vi "setEndLabel.vi"(0 "reference":refnum<class "SegmentedLineEdge.lvclass">, 1 "endLabel":string, 5 "error in (no error)":errorcluster) -> (14 "reference out":refnum<class "SegmentedLineEdge.lvclass">, 19 "error out":errorcluster)   [LabVIEW 2016, in "SegmentedLineEdge.lvclass"]
doc: "public void setEndLabel(String newValue)"
uses:
  <resource>/Framework/Providers/Open_GDS/UML/SegmentedLineEdge_class/SegmentedLineEdge.lvclass
panel:
  # "Always set\nVI Server class\nto current VI. Do not\nconnect this control\nto the connector pane.\n(Tip!: Just drag\nand drop the icon\ninto the refnum)"
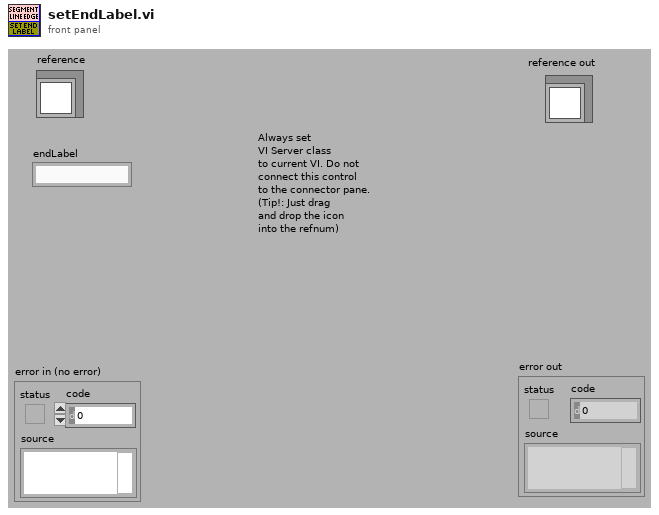
[diagram p1: front panel]
types:
  T1 = typedef "SegmentedLineEdge.lvclass/ObjectAttributes.ctl" = cluster{"lineStyle":refnum<class "LineStyle.lvclass">, "startArrowHead":refnum<class "ArrowHead.lvclass">, "endArrowHead":refnum<class "ArrowHead.lvclass">, "startLabel":string, "midLabel":string, "endLabel":string, "MidLabelOffset":T2, "SplitWire":bool}
  T2 = typedef "Point Point2D.ctl" = cluster{"x":dbl, "y":dbl}
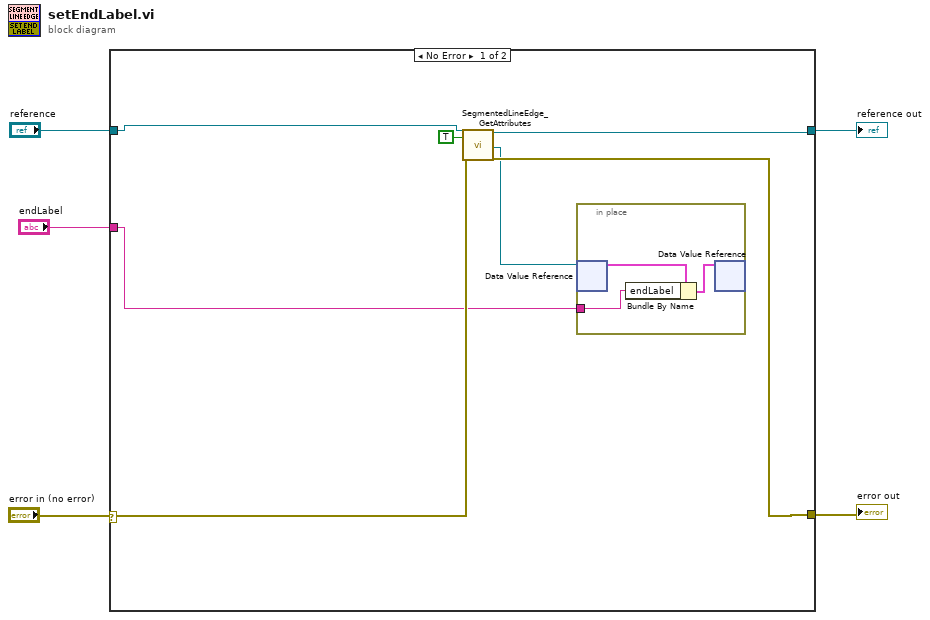
[diagram p0: block diagram]
diagram:
  n1 = case shown="No Error" "error in (no error)" {
    selector: "error in (no error)" -> [w9 w16]
    tunnel: "reference" -> [w12 w17]
    tunnel: [w11 w16] -> w4
    tunnel: [w10 w17] -> w3
    tunnel: "endLabel" -> [w6 _]
    frame No Error {
      n2 = call <resource>:"SegmentedLineEdge_GetAttributes.vi"("reference in"=w12, "OnlyGetDvrReference(False)"=TRUE, "error in (no error)"=w9) -> ("reference out"=w10:refnum<class "SegmentedLineEdge.lvclass">, "DataRef"=w7:refnum<data-value>, "error out"=w11:errorcluster)  [unwired: 13 in, 1 out]
      n3 = in-place {
        in-place-border: w6 -> [w14]
        n4 = in-place-dvr #1(w7) -> (w15:T1)  [unwired: 1 out]
        n5 = Bundle By Name(cluster=w15, "endLabel"=w14) -> (w13:T1)
        n6 = in-place-dvr #1(w13) -> ()  [unwired: 2 out]
      }
    }
    frame Error {
    }
  }
  "reference out" <- w3
  "error out" <- w4
